vi "Delete FPGA Addon.vi"(8 "error in (no error)":errorcluster, 11 "FPGA Addon refnum":T1=18446744073709551615 format="%.0x") -> (0 "error out":errorcluster, 2 "Deleted?":bool)   [LabVIEW 2018, in "Scripting API.lvlib"]
uses:
  Scripting API.lvlib
  <vilib>/NI Veristand/Custom Device API/Custom Device Item Ref.ctl
  <vilib>/NI Veristand/Custom Device API/Custom Device API.lvlib
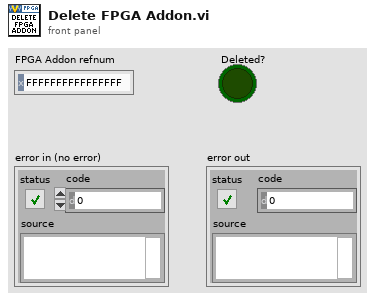
[diagram p1: front panel]
types:
  T1 = typedef "Custom Device API.lvlib/Custom Device Item Ref.ctl" = u64
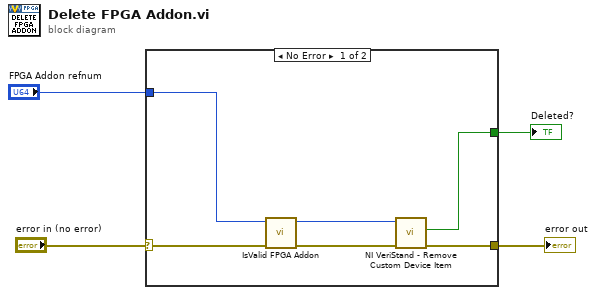
[diagram p0: block diagram]
diagram:
  n1 = case shown="No Error" "error in (no error)" {
    selector: "error in (no error)" -> [w9 w11]
    tunnel: [w10 w11] -> w4
    tunnel: "FPGA Addon refnum" -> [w8 _]
    tunnel: [w5 _] -> w1
    frame No Error {
      n2 = call "IsValid FPGA Addon.vi"("error in (no error)"=w9, "FPGA Addon refnum in"=w8) -> ("error out"=w6:errorcluster, "FPGA Addon refnum out"=w7:T1)  [unwired: 8 in]
      n3 = call <vilib>:"NI VeriStand - Remove Custom Device Item.vi"("error in (no error)"=w6, "Item Ref in"=w7) -> ("error out"=w10:errorcluster, "Deleted?"=w5:bool)  [unwired: 8 in]
    }
    frame Error {
    }
  }
  "error out" <- w4
  "Deleted?" <- w1
